vi "LakeShore350Full.vi"() -> ()   [LabVIEW 2015]
uses:
  SECoP.lvlib
  <vilib>/regexp/Match Regular Expression.xnode
  Program Files (x86)/National Instruments/LabVIEW 2016/instr.lib/Lake Shore 350/Lake Shore 350.lvlib
  Program Files (x86)/National Instruments/LabVIEW 2016/instr.lib/Lake Shore 350/Public/Data/Sensor Data (Single Reading).vi
  parametertype.ctl
panel:
  out "error out":errorcluster
  out "log":string
  in  "DLL path":path=path "C:/Users/user/Desktop/x86_32"
  in  "stop":bool
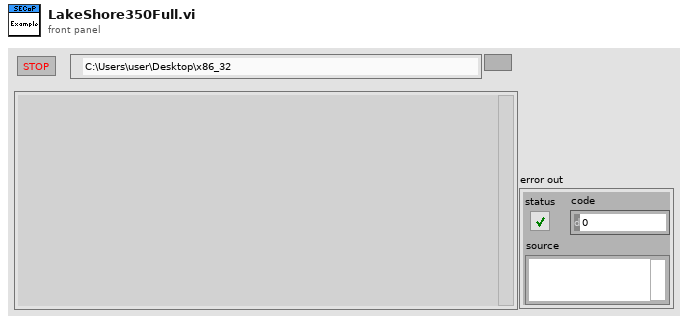
[diagram p1: front panel]
types:
  T1 = typedef "parametertype.ctl" = enum8{"readonly", "readwrite", "command"}
  T2 = cluster{"name":string, "type":T1, "datatype":string, "description":string}[]
  T3 = cluster{"Baud Rate":u32, "Parity":u16, "Data Bits":u16, "Stop Bits":u16, "Flow Control":u16}
  T4 = typedef "SECoP.lvlib/SECoP-libraries.ctl" = cluster{"serverDLL":path, "variantDLL":path, "cleanup_mode":bool}
  T5 = typedef "SECoP.lvlib/SECoP-action.ctl" = enum32{"any action", "read", "change", "do cmd"}
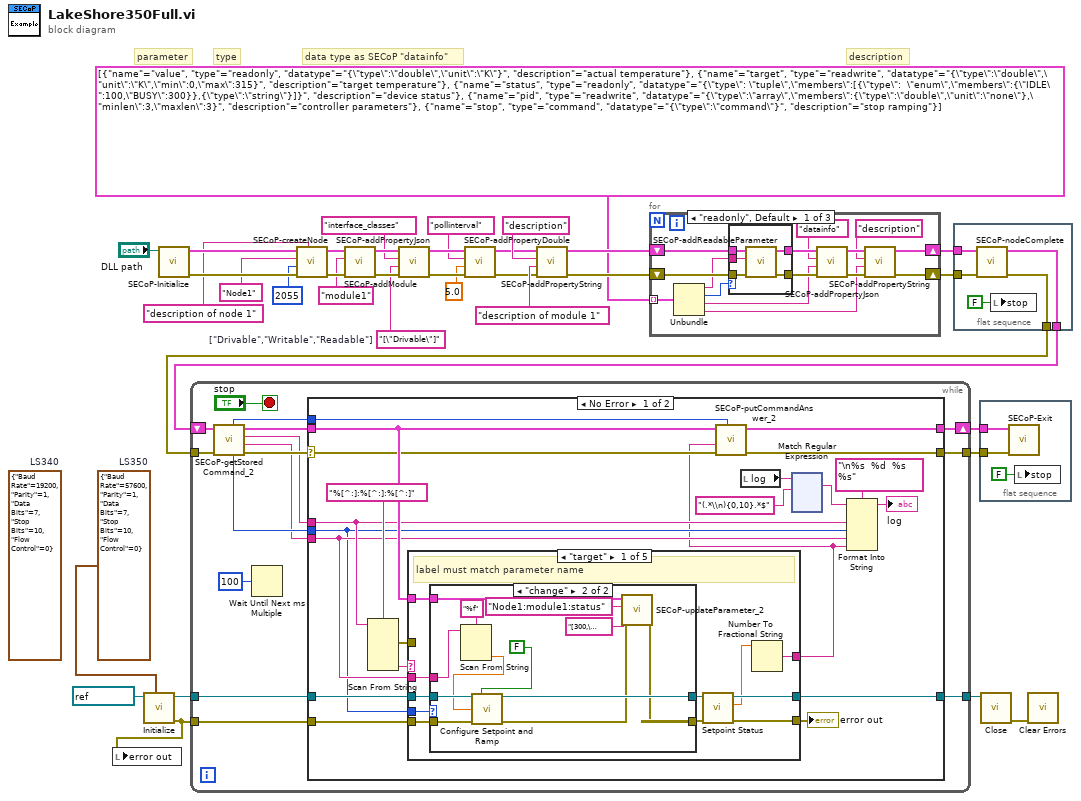
[diagram p0: block diagram]
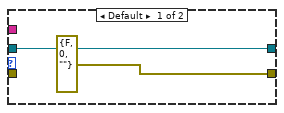
[diagram p2: hidden frame]
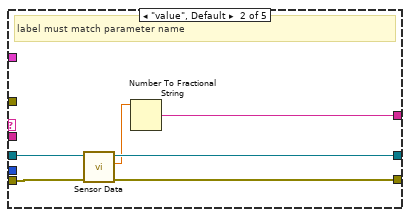
[diagram p3: hidden frame]
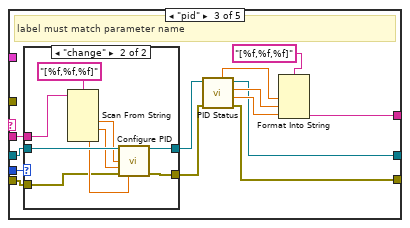
[diagram p4: hidden frame]
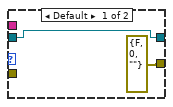
[diagram p5: hidden frame]
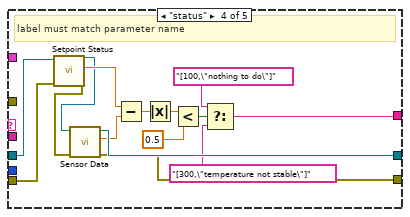
[diagram p6: hidden frame]
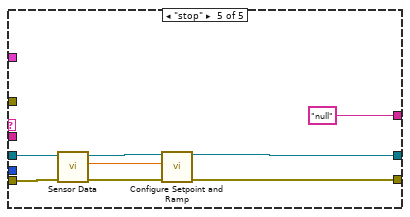
[diagram p7: hidden frame]
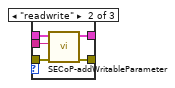
[diagram p9: hidden frame]
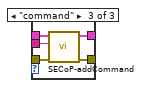
[diagram p10: hidden frame]
diagram:
  (unwired) T3 {"Baud Rate"=19200, "Parity"=1, "Data Bits"=7, "Stop Bits"=10, "Flow Control"=0}  # LS340
  w2 = T3 {"Baud Rate"=57600, "Parity"=1, "Data Bits"=7, "Stop Bits"=10, "Flow Control"=0}  # LS350
  w24 = "[\"Drivable\"]"  # ["Drivable","Writable","Readable"]
  # "description"
  # "data type as SECoP \"datainfo\""
  # "type"
  # "parameter"
  n1 = call "Initialize.vi"("Serial Configuration"=w2, "VISA resource name"=refnum<visa-resource-name> "COM4") -> ("error out"=w3:errorcluster, "VISA resource name out"=w6:refnum<visa-resource-name>)  [unwired: 8 in]
  n2 = local write "error out"(w3) -> ()
  n3 = call "SECoP-Initialize.vi"("DLL path (in)"="DLL path") -> ("error out"=w34:errorcluster, "DLL path (out)"=w35:T4)  [unwired: 9 in]
  n4 = while {
    shift-right: [w51] -> w23
    shift-left: w10 -> [w49]
    tunnel: w11 -> [w48]
    tunnel: [w41] -> w22
    tunnel: w6 -> [w39]
    tunnel: [w38] -> w5
    tunnel: w3 -> [w37]
    stop <- "stop" stop-if-true
    n5 = call "SECoP-getStoredCommand_2.vi"("error in (no error)"=w48, "DLL path (in)"=w49) -> ("error out"=w46:errorcluster, "arguments/setvalue"=w42:string, "command/parameter path"=w43:string, "DLL path (out)"=w47:T4, "action"=w44:T5, "command id"=w45:u64)  [unwired: 4 in]
    n6 = Wait Until Next ms Multiple(millisecond multiple=u32 100) -> ()  [unwired: 1 out]
    n7 = case shown="No Error" w46 {
      selector: w46 -> [w71 w266]
      tunnel: w47 -> [w72 w267]
      tunnel: [w70 w267] -> w51
      tunnel: w45 -> [w69 _]
      tunnel: w43 -> [w62 _]
      tunnel: w42 -> [w58 _]
      tunnel: w44 -> [w57 _]
      tunnel: [w68 w266] -> w41
      tunnel: w39 -> [w59 w265]
      tunnel: [w56 w265] -> w38
      tunnel: w37 -> [w54 _]
      frame No Error {
        n8 = Scan From String(format string="%[^:]:%[^:]:%[^:]", input string=w62) -> (error out=w61:errorcluster, output 3=w52:string)  [unwired: 7 in, 2 out]
        n9 = case shown="\"target\"" w52 {
          tunnel: [w74 w102 w109 w132 "null"] -> w53
          tunnel: w61 -> [_ _ _ _ _]
          tunnel: w59 -> [w82 w103 w115 w141 w149]
          tunnel: w58 -> [w83 _ w114 _ _]
          tunnel: [w78 w101 w104 w142 w145] -> w56
          tunnel: w57 -> [w81 _ w116 _ _]
          tunnel: [w79 w100 w108 w130 w144] -> w55
          tunnel: w54 -> [w80 w99 w113 w128 w150]
          tunnel: w72 -> [w73 _ _ _ _]
          frame "target" {
            # "label must match parameter name"
            n10 = case shown="\"change\"" w81 {
              tunnel: w83 -> [_ w95]
              tunnel: w82 -> [w85 w97]
              tunnel: [errorcluster {"status"=FALSE, "code"=0, "source"=""} ("error out") w88] -> w77
              tunnel: [w85 w96] -> w76
              tunnel: w80 -> [_ w93]
              tunnel: w73 -> [_ w90]
              frame Default {
              }
              frame "change" {
                n11 = Scan From String(format string="%f", input string=w95) -> (output 1=w92:dbl)  [unwired: 3 in, 3 out]
                n12 = call "Configure Setpoint and Ramp.vi"("VISA resource name"=w97, "Enable Setpoint Ramping  (F: Disable)"=FALSE, "Setpoint (0.00000)"=w92, "error in (no error)"=w93) -> ("VISA resource name out"=w96:refnum<visa-resource-name>, "error out"=w89:errorcluster)  [unwired: 10 in]
                n13 = call "SECoP-updateParameter_2.vi"("error in (no error)"=w89, "value"="[300,\"temperature not stable\"]" ("Value"), "parameter name"="Node1:module1:status" ("Parameter name"), "DLL path (in)"=w90) -> ("error out"=w88:errorcluster)  [unwired: 6 in, 1 out]
              }
            }
            n14 = call "Setpoint Status.vi"("error in (no error)"=w77, "VISA resource name"=w76) -> ("error out"=w79:errorcluster, "Setpoint"=w75:dbl, "VISA resource name out"=w78:refnum<visa-resource-name>)  [unwired: 7 in]
            n15 = Number To Fractional String(number=w75) -> (F-format string=w74:string)  [unwired: 3 in]
          }
          frame "value", Default {
            # "label must match parameter name"
            n16 = call-poly "Sensor Data.vi"("error in (no error)"=w99, "VISA resource name"=w103) -> ("error out"=w100:errorcluster, "Sensor Data"=w98:dbl, "VISA resource name out"=w101:refnum<visa-resource-name>)  [unwired: 7 in]
            n17 = Number To Fractional String(number=w98) -> (F-format string=w102:string)  [unwired: 3 in]
          }
          frame "pid" {
            # "label must match parameter name"
            n18 = case shown="\"change\"" w116 {
              tunnel: w115 -> [w118 w127]
              tunnel: w114 -> [_ w122]
              tunnel: [w118 w121] -> w105
              tunnel: [errorcluster {"status"=FALSE, "code"=0, "source"=""} ("error out") w120] -> w106
              tunnel: w113 -> [_ w119]
              frame Default {
              }
              frame "change" {
                n19 = Scan From String(format string="[%f,%f,%f]", input string=w122) -> (output 1=w125:dbl, output 2=w124:dbl, output 3=w123:dbl)  [unwired: 5 in, 3 out]
                n20 = call "Configure PID.vi"("VISA resource name"=w127, "Gain (P) (50.0)"=w125, "Reset (I) (20.0)"=w124, "error in (no error)"=w119, "Rate (D) (0.0 %)"=w123) -> ("VISA resource name out"=w121:refnum<visa-resource-name>, "error out"=w120:errorcluster)  [unwired: 9 in]
              }
            }
            n21 = call "PID Status.vi"("error in (no error)"=w106, "VISA resource name"=w105) -> ("error out"=w108:errorcluster, "Rate (D)"=w112:dbl, "Reset (I)"=w110:dbl, "VISA resource name out"=w104:refnum<visa-resource-name>, "Gain (P)"=w111:dbl)  [unwired: 5 in]
            n22 = Format Into String(format string="[%f,%f,%f]", w111, w110, w112) -> (resulting string=w109:string)  [unwired: 2 in, 1 out]
          }
          frame "status" {
            # "label must match parameter name"
            n23 = call "Setpoint Status.vi"("error in (no error)"=w128, "VISA resource name"=w141) -> ("error out"=w131:errorcluster, "Setpoint"=w140:dbl, "VISA resource name out"=w129:refnum<visa-resource-name>)  [unwired: 7 in]
            n24 = call-poly "Sensor Data.vi"("error in (no error)"=w131, "VISA resource name"=w129) -> ("error out"=w130:errorcluster, "Sensor Data"=w139:dbl, "VISA resource name out"=w142:refnum<visa-resource-name>)  [unwired: 7 in]
            n25 = Subtract(x=w140, y=w139) -> (x-y=w138:dbl)
            n26 = Absolute Value(x=w138) -> (abs(x)=w137:dbl)
            n27 = Less?(x=w137, y=0.5) -> (x < y?=w135:bool)
            n28 = Select(t="[100,\"nothing to do\"]", s=w135, f="[300,\"temperature not stable\"]") -> (s? t:f=w132:string)
          }
          frame "stop" {
            n29 = call-poly "Sensor Data.vi"("error in (no error)"=w150, "VISA resource name"=w149) -> ("error out"=w148:errorcluster, "Sensor Data"=w146:dbl, "VISA resource name out"=w147:refnum<visa-resource-name>)  [unwired: 7 in]
            n30 = call "Configure Setpoint and Ramp.vi"("VISA resource name"=w147, "Setpoint (0.00000)"=w146, "error in (no error)"=w148) -> ("VISA resource name out"=w145:refnum<visa-resource-name>, "error out"=w144:errorcluster)  [unwired: 11 in]
          }
        }
        "error out" <- w55
        n31 = call "SECoP-putCommandAnswer_2.vi"("command id"=w69, "error in (no error)"=w71, "value"=w53, "DLL path (in)"=w72) -> ("error out"=w68:errorcluster, "DLL path (out)"=w70:T4)  [unwired: 6 in]
        n32 = local read "log"() -> (w65:string)
        n33 = xnode "Match Regular Expression"("input string"=w65, "regular expression"="(.*\\n){0,10}.*$") -> ("whole match"=w66:string)  [unwired: 4 in, 4 out]
        n34 = Format Into String(format string="\n%s  %d  %s  %s", initial string=w66, w62, w57, w58, w53) -> (resulting string=→"log":string)  [unwired: 1 in, 1 out]
      }
      frame Error {
      }
    }
  }
  n35 = call "SECoP-createNode.vi"("description"="description of node 1", "error in (no error)"=w34, "TCP port"=u16 2055, "node id"="Node1" ("id"), "DLL path (in)"=w35) -> ("error out"=w29:errorcluster, "DLL path (out)"=w33:T4)  [unwired: 5 in]
  n36 = call "SECoP-addModule.vi"("error in (no error)"=w29, "module name"="module1" ("name"), "DLL path (in)"=w33) -> ("error out"=w26:errorcluster, "DLL path (out)"=w27:T4)  [unwired: 7 in]
  n37 = call "SECoP-addPropertyJson.vi"("error in (no error)"=w26, "property value"=w24, "property name"="interface_classes" ("name"), "DLL path (in)"=w27) -> ("error out"=w15:errorcluster, "DLL path (out)"=w17:T4)  [unwired: 6 in]
  n38 = call "SECoP-addPropertyDouble.vi"("error in (no error)"=w15, "property value"=5.0, "property name"="pollinterval", "DLL path (in)"=w17) -> ("error out"=w14:errorcluster, "DLL path (out)"=w16:T4)  [unwired: 6 in]
  n39 = call "SECoP-addPropertyString.vi"("error in (no error)"=w14, "property value"="description of module 1" ("name"), "property name"="description" ("name"), "DLL path (in)"=w16) -> ("error out"=w20:errorcluster, "DLL path (out)"=w21:T4)  [unwired: 6 in]
  n40 = for {
    tunnel: T2 [{"name"="value", "type"=enum."readonly", "datatype"="{\"type\":\"double\",\"unit\":\"K\"}", "description"="actual temperature"}, {"name"="target", "type"=enum."readwrite", "datatype"="{\"type\":\"double\",\"unit\":\"K\",\"min\":0,\"max\":315}", "description"="target temperature"}, {"name"="status", "type"=enum."readonly", "datatype"="{\"type\": \"tuple\",\"members\":[{\"type\":  \"enum\",\"members\":{\"IDLE\":100,\"BUSY\":300}},{\"type\":\"string\"}]}", "description"="device status"}, {"name"="pid", "type"=enum."readwrite", "datatype"="{\"type\":\"array\",\"members\":{\"type\":\"double\",\"unit\":\"none\"},\"minlen\":3,\"maxlen\":3}", "description"="controller parameters"}, {"name"="stop", "type"=enum."command", "datatype"="{\"type\":\"command\"}", "description"="stop ramping"}] -> [w270] mode=indexing
    shift-right: [w269] -> w9
    shift-left: w21 -> [w279]
    shift-right: [w268] -> w8
    shift-left: w20 -> [w278]
    n41 = Unbundle(w270) -> ("name"=w271:string, "type"=w280:T1, "datatype"=w272:string, "description"=w273:string)
    n42 = case shown="\"readonly\", Default" w280 {
      tunnel: w271 -> [w285 w292 w297]
      tunnel: w279 -> [w287 w291 w296]
      tunnel: [w286 w290 w295] -> w277
      tunnel: [w283 w288 w293] -> w276
      tunnel: w278 -> [w284 w289 w294]
      frame "readonly", Default {
        n43 = call "SECoP-addReadableParameter.vi"("error in (no error)"=w284, "parameter name"=w285, "DLL path (in)"=w287) -> ("error out"=w283:errorcluster, "DLL path (out)"=w286:T4)  [unwired: 7 in]
      }
      frame "readwrite" {
        n44 = call "SECoP-addWritableParameter.vi"("error in (no error)"=w289, "parameter name"=w292, "DLL path (in)"=w291) -> ("error out"=w288:errorcluster, "DLL path (out)"=w290:T4)  [unwired: 7 in]
      }
      frame "command" {
        n45 = call "SECoP-addCommand.vi"("error in (no error)"=w294, "command name"=w297, "DLL path (in)"=w296) -> ("error out"=w293:errorcluster, "DLL path (out)"=w295:T4)  [unwired: 7 in]
      }
    }
    n46 = call "SECoP-addPropertyJson.vi"("error in (no error)"=w276, "property value"=w272, "property name"="datainfo" ("name"), "DLL path (in)"=w277) -> ("error out"=w281:errorcluster, "DLL path (out)"=w282:T4)  [unwired: 6 in]
    n47 = call "SECoP-addPropertyString.vi"("error in (no error)"=w281, "property value"=w273, "property name"="description" ("name"), "DLL path (in)"=w282) -> ("error out"=w268:errorcluster, "DLL path (out)"=w269:T4)  [unwired: 6 in]
  }
  n48 = flat-sequence {
    tunnel: w9 -> [w301]
    tunnel: w8 -> [w300]
    tunnel: [w298] -> w10
    tunnel: [w299] -> w11
    frame #0 {
      n49 = call "SECoP-nodeComplete.vi"("error in (no error)"=w300, "DLL path (in)"=w301) -> ("error out"=w299:errorcluster, "DLL path (out)"=w298:T4)  [unwired: 8 in]
      n50 = local write "stop"(FALSE) -> ()
    }
  }
  n51 = flat-sequence {
    tunnel: w23 -> [w304]
    tunnel: w22 -> [w303]
    frame #0 {
      n52 = call "SECoP-Exit.vi"("error in (no error)"=w303, "DLL path (in)"=w304) -> ()  [unwired: 9 in, 1 out]
      n53 = local write "stop"(FALSE) -> ()
    }
  }
  n54 = call "Close.vi"("VISA resource name"=w5) -> ("error out"=w4:errorcluster)  [unwired: 10 in]
  n55 = call <vilib>:"Clear Errors.vi"("error in (no error)"=w4) -> ()  [unwired: 5 in, 2 out]
